vi "Actor Core.vi"(8 "error in":errorcluster, 11 "GRMActor in":refnum<class "GeneralRMActor.lvclass">) -> (0 "error out":errorcluster, 3 "Actor out":refnum<class "Actor.lvclass">)   [LabVIEW 2020, in "GeneralRMActor.lvlib" / "GeneralRMActor.lvclass"]
doc: "(<B>Filename</B>: Actor Framework.lvlib:Actor.lvclass:Actor Core.vi)\n\nReceives messages to the actor, reacts to them, and initiates any error handling that may shut the actor down.\n\nDescendant classes may override this VI to append parallel tasks for the actor to complete while it handles messages. Overrides use the Call Parent Class Method node."
uses:
  GeneralRMActor.lvclass
  <vilib>/ActorFramework/Actor/Actor.lvclass
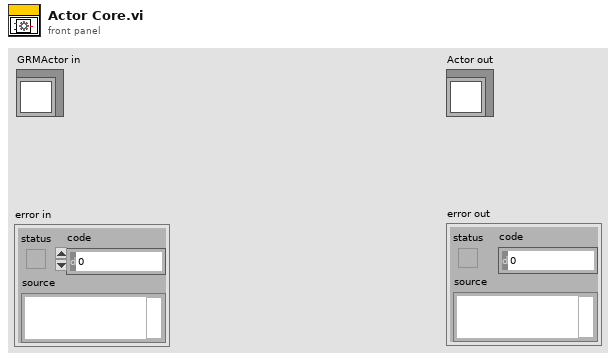
[diagram p1: front panel]
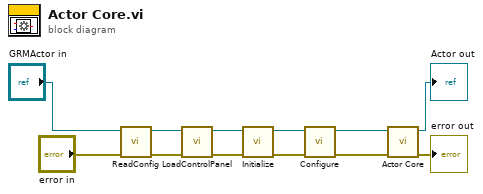
[diagram p0: block diagram]
diagram:
  n1 = call-dynamic "ReadConfig.vi"("error in (no error)"="error in", "GRMActor in"="GRMActor in") -> ("error out"=w9:errorcluster, "GRMActor out"=w6:refnum<class "GeneralRMActor.lvclass">)  [unwired: 8 in]
  n2 = call-dynamic "LoadControlPanel.vi"("error in (no error)"=w9, "GRMActor in"=w6) -> ("error out"=w7:errorcluster, "GRMActor out"=w4:refnum<class "GeneralRMActor.lvclass">)  [unwired: 8 in]
  n3 = call-dynamic "Initialize.vi"("error in (no error)"=w7, "GRMActor in"=w4) -> ("error out"=w5:errorcluster, "GRMActor out"=w2:refnum<class "GeneralRMActor.lvclass">)  [unwired: 8 in]
  n4 = call-dynamic "Configure.vi"("error in (no error)"=w5, "GRMActor in"=w2) -> ("error out"=w3:errorcluster, "GRMActor out"=w1:refnum<class "GeneralRMActor.lvclass">)  [unwired: 8 in]
  n5 = call-parent "Actor Core.vi"("error in"=w3, "Actor in"=w1) -> ("error out"=→"error out":errorcluster, "Actor out"=→"Actor out":refnum<class "Actor.lvclass">)  [unwired: 8 in]
